vi "Add.vi"(8 "error in":errorcluster, 9 "Y":i32, 10 "X":i32, 11 "Uno in":refnum<class "Uno.lvclass">) -> (0 "error out":errorcluster, 3 "Uno out":refnum<class "Uno.lvclass">)   [LabVIEW 2020, in "Uno.lvclass"]
uses:
  Uno.lvclass
  Uno.lvclass/Uno.ctl
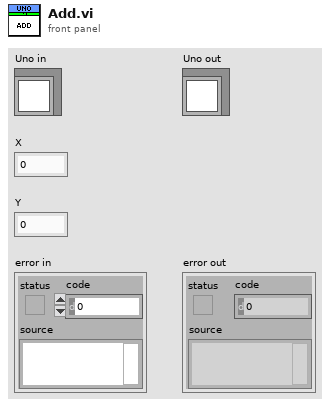
[diagram p1: front panel]
types:
  T1 = typedef "Uno.lvclass/Group Data.ctl" = cluster{"our positions":u8[][]}
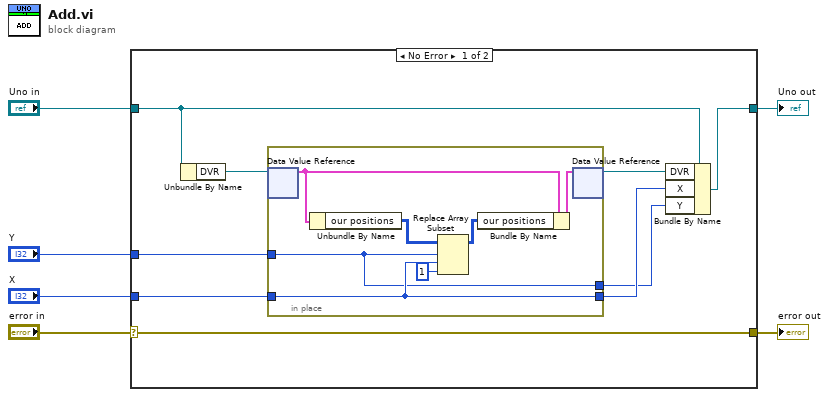
[diagram p0: block diagram]
diagram:
  n1 = case shown="No Error" "error in" {
    selector: "error in" -> [w15 w24]
    tunnel: [w15 w24] -> w5
    tunnel: [w13 w23] -> w3
    tunnel: "Uno in" -> [w14 w23]
    tunnel: "Y" -> [w10 _]
    tunnel: "X" -> [w9 _]
    frame No Error {
      n2 = Unbundle By Name(w14) -> ("DVR"=w11:refnum<data-value>)
      n3 = in-place {
        in-place-border: w10 -> [w17]
        in-place-border: w9 -> [w18]
        in-place-border: [w18] -> w8
        in-place-border: [w17] -> w7
        n4 = in-place-dvr #1(w11) -> (w22:T1)  [unwired: 1 out]
        n5 = Unbundle By Name(w22) -> ("our positions"=w20:u8[][])
        n6 = Replace Array Subset(array=w20, new element=u8 1 ("new element/subarray"), index (row)=w17, index (col)=w18) -> (w19:u8[][])
        n7 = Bundle By Name(cluster=w22, "our positions"=w19) -> (w21:T1)
        n8 = in-place-dvr #1(w21) -> (w12:refnum<data-value>)  [unwired: 1 out]
      }
      n9 = Bundle By Name(cluster=w14, "DVR"=w12, "X"=w8, "Y"=w7) -> (w13:refnum<class "Uno.lvclass">)
    }
    frame Error {
    }
  }
  "error out" <- w5
  "Uno out" <- w3
